vi "Joystick and Camera SHIH V5- external Connection.vi"(0 "Motion in":refnum<class "Motion.lvclass">, 1 "XYZTheta":dbl[](array[numeric])=[584.964, 676.042, 69.3079, 0.000384], 2 "Measurement Point":string, 3 "Inital GO":bool=TRUE) -> (5 "final out":dbl[](array[numeric]), 7 "Motion out":refnum<class "Motion.lvclass">, 10 "error out":errorcluster)   [LabVIEW 2016]
uses:
  Classes/Controllers/Motion/Copy of Motion Folder/Motion.lvclass
panel:
  in  "how many times per measurement":dbl=50.0
  out "Gantry position":dbl[](array[numeric])
  in  "start measurement":bool
  in  "Joystick":bool
  in  "Stop":bool
  # "new world"
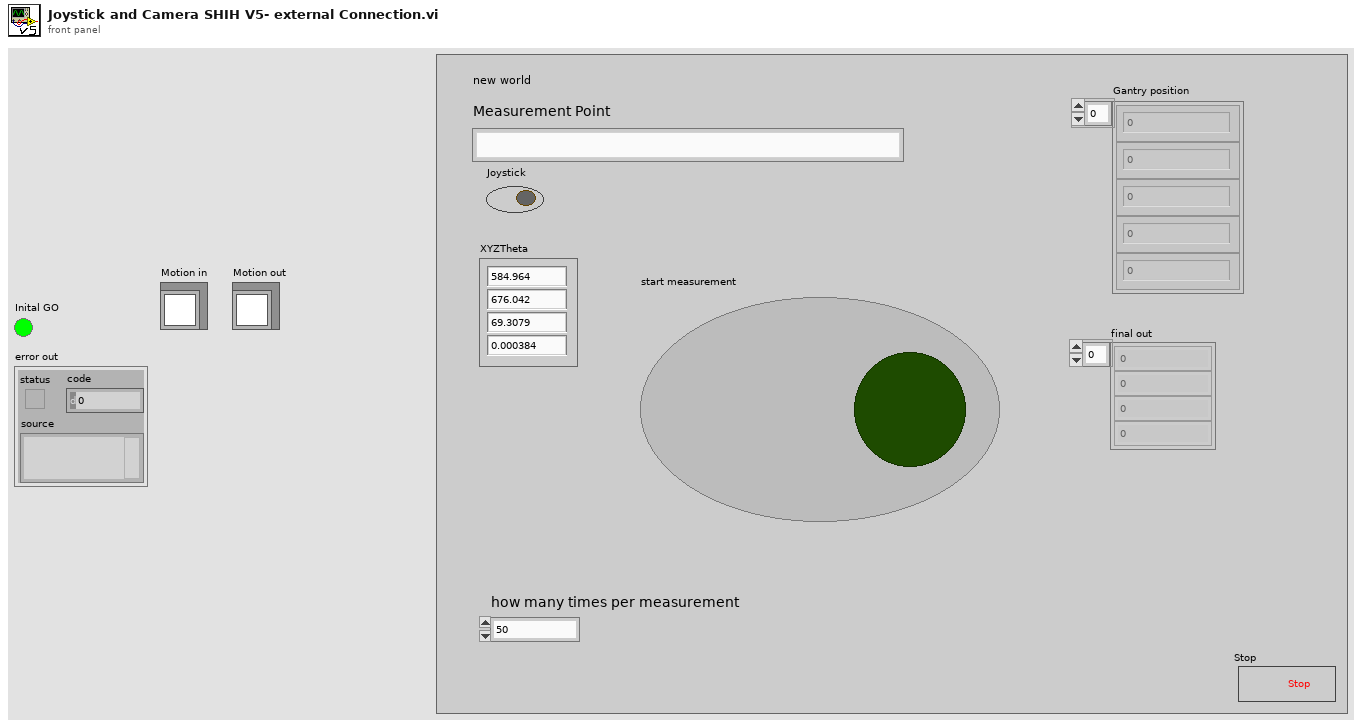
[diagram p1: front panel]
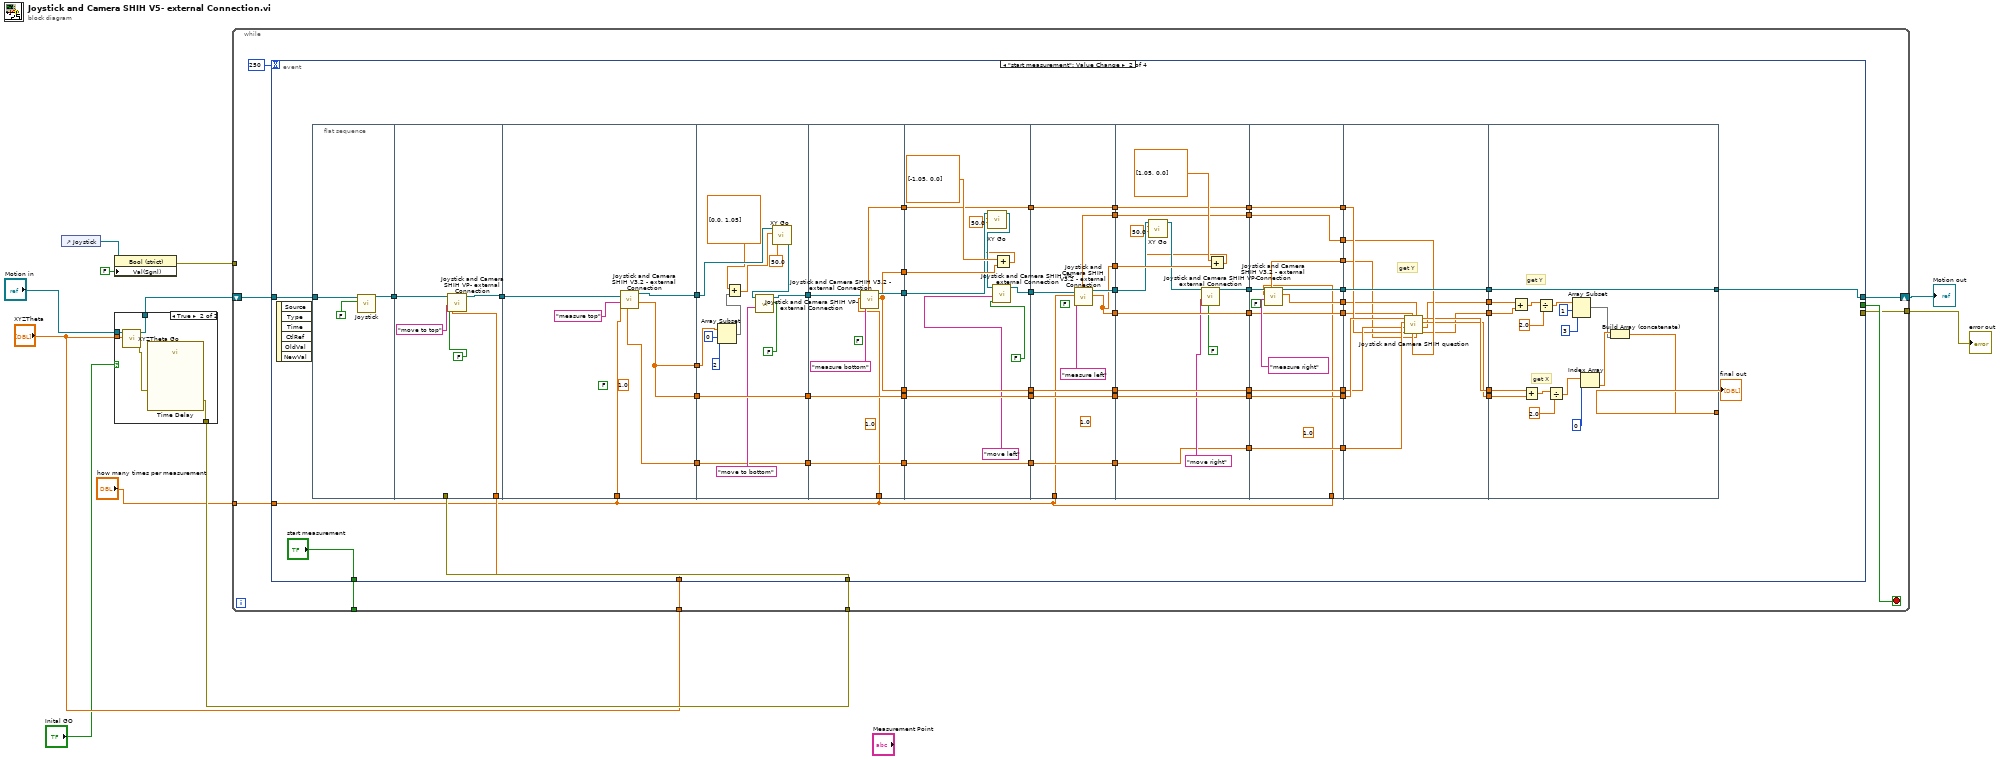
[diagram p0: block diagram]
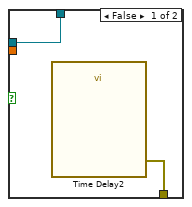
[diagram p2: hidden frame]
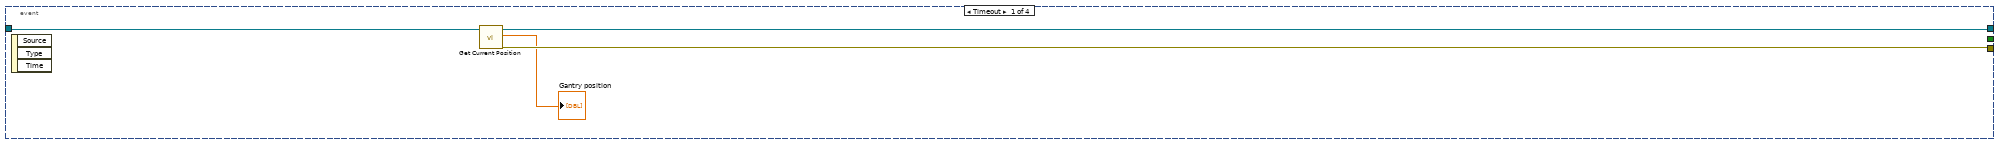
[diagram p3: hidden frame]
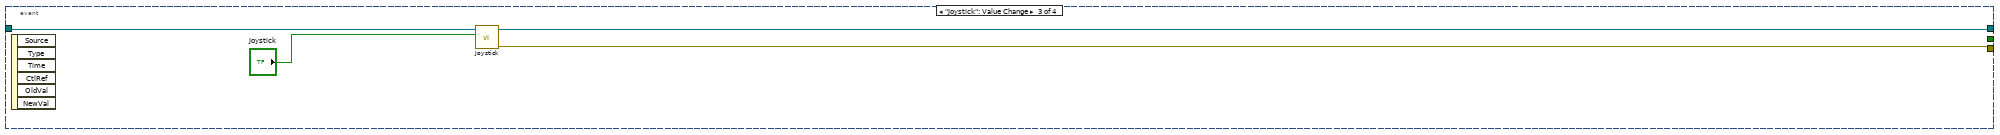
[diagram p4: hidden frame]
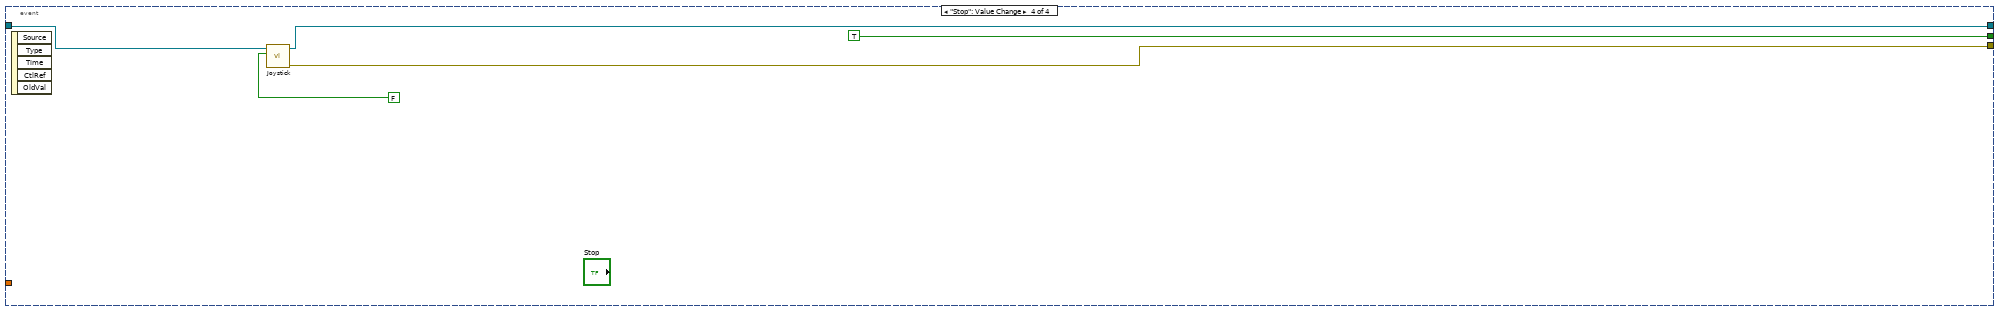
[diagram p5: hidden frame]
diagram:
  n1 = control-ref of="Joystick"() -> (w10:refnum<vi>)
  n2 = case shown="True" "Inital GO" {
    tunnel: "Motion in" -> [w13 w18]
    tunnel: [w13 w17] -> w5
    tunnel: [w12 w15] -> w4
    tunnel: "XYZTheta" -> [_ w14]
    frame False {
      n3 = call "Time Delay2"() -> ("error out"=w12:errorcluster)  [unwired: 11 in]
    }
    frame True {
      n4 = call "XYZTheta Go.vi"("XYZTheta In"=w14, "Motion in"=w18) -> ("error out"=w16:errorcluster, "Motion out"=w17:refnum<class "Motion.lvclass">)  [unwired: 7 in, 1 out]
      n5 = call "Time Delay"("error in (no error)"=w16) -> ("error out"=w15:errorcluster)  [unwired: 10 in]
    }
  }
  n6 = property class="Bool (strict)"(reference=w10, "Val(Sgnl)"=FALSE ("Value (Signaling)")) -> (error out=w9:errorcluster)  [unwired: 1 in, 1 out]
  n7 = while {
    shift-right: [w24] -> w8
    shift-left: w5 -> [w25]
    tunnel: w9 -> [_]
    tunnel: [w23] -> w7
    tunnel: w4 -> [w22]
    tunnel: "XYZTheta" -> [w21]
    tunnel: [w20] -> _
    tunnel: "how many times per measurement" -> [w19]
    stop <- w26 stop-if-true
    n8 = event shown="[1] \"start measurement\": Value Change" {
      selector: _ -> [_ _ _ _]
      dyn-events: _ -> [_ _ _ _]
      timeout: 250 -> [_ _ _ _]
      tunnel: [_ _ _ TRUE] -> w26
      tunnel: w25 -> [w31 w87 w207 w211]
      tunnel: [w30 w62 w205 w210] -> w24
      tunnel: [w29 _ w204 w208] -> w23
      tunnel: w22 -> [_ w86 _ _]
      tunnel: w21 -> [_ w64 _ _]
      tunnel: [_ "start measurement" _ _] -> w20
      tunnel: w19 -> [_ w32 _ _]
      event Timeout {
        n9 = event-data() -> ()  [unwired: 1 in, 3 out]
        n10 = call-dynamic "Get Current Position.vi"("Motion in"=w31) -> ("error out"=w29:errorcluster, "XYZTheta Out"=→"Gantry position":dbl[], "Motion out"=w30:refnum<class "Motion.lvclass">)  [unwired: 8 in]
      }
      event "start measurement": Value Change {
        n11 = event-data() -> ()  [unwired: 1 in, 6 out]
        n12 = flat-sequence {
          tunnel: w87 -> [w89]
          tunnel: [w88] -> w84
          tunnel: w86 -> [_]
          tunnel: [w91] -> w85
          tunnel: w84 -> [w95]
          tunnel: w64 -> [w92]
          tunnel: w85 -> [w101]
          tunnel: [w100] -> w83
          tunnel: [w98] -> w72
          tunnel: [w98] -> w61
          tunnel: [w97] -> w48
          tunnel: w32 -> [w96]
          tunnel: w83 -> [w111]
          tunnel: [w114] -> w82
          tunnel: [w115] -> w73
          tunnel: w72 -> [w115]
          tunnel: w61 -> [w106]
          tunnel: w48 -> [w102]
          tunnel: [w102] -> w47
          tunnel: w82 -> [w123]
          tunnel: [w121] -> w81
          tunnel: [w120] -> w74
          tunnel: w73 -> [w120]
          tunnel: [w119] -> w68
          tunnel: [w119] -> w60
          tunnel: w47 -> [w118]
          tunnel: [w118] -> w46
          tunnel: [w117] -> w41
          tunnel: w32 -> [w116]
          tunnel: w81 -> [w129]
          tunnel: [w134] -> w80
          tunnel: [w136] -> w75
          tunnel: w74 -> [w136]
          tunnel: [w135] -> w69
          tunnel: w68 -> [w135]
          tunnel: w60 -> [w130]
          tunnel: w46 -> [w125]
          tunnel: [w125] -> w45
          tunnel: w41 -> [w124]
          tunnel: [w124] -> w40
          tunnel: w80 -> [w146]
          tunnel: [w145] -> w79
          tunnel: [w143] -> w76
          tunnel: w75 -> [w143]
          tunnel: [w142] -> w70
          tunnel: w69 -> [w142]
          tunnel: [w141] -> w66
          tunnel: [w141] -> w59
          tunnel: w45 -> [w140]
          tunnel: [w140] -> w44
          tunnel: w40 -> [w139]
          tunnel: [w139] -> w39
          tunnel: [w138] -> w36
          tunnel: w32 -> [w137]
          tunnel: w79 -> [w153]
          tunnel: [w158] -> w78
          tunnel: [w161] -> w77
          tunnel: w76 -> [w161]
          tunnel: [w160] -> w71
          tunnel: w70 -> [w160]
          tunnel: [w159] -> w67
          tunnel: w66 -> [w159]
          tunnel: w59 -> [w154]
          tunnel: w44 -> [w149]
          tunnel: [w149] -> w43
          tunnel: w39 -> [w148]
          tunnel: [w148] -> w38
          tunnel: w36 -> [w147]
          tunnel: [w147] -> w35
          tunnel: w78 -> [w173]
          tunnel: [w171] -> w58
          tunnel: w77 -> [w171]
          tunnel: [w170] -> w56
          tunnel: w71 -> [w170]
          tunnel: [w169] -> w54
          tunnel: [w168] -> w52
          tunnel: w67 -> [w168]
          tunnel: [w167] -> w50
          tunnel: w43 -> [w166]
          tunnel: [w166] -> w42
          tunnel: w38 -> [w165]
          tunnel: [w165] -> w37
          tunnel: w35 -> [w164]
          tunnel: [w164] -> w34
          tunnel: [w163] -> w33
          tunnel: w32 -> [w162]
          tunnel: w58 -> [w185]
          tunnel: [w176] -> w57
          tunnel: w56 -> [w183]
          tunnel: [w177] -> w55
          tunnel: w54 -> [w179]
          tunnel: [w175] -> w53
          tunnel: w52 -> [w181]
          tunnel: [w174] -> w51
          tunnel: w50 -> [w186]
          tunnel: [w186] -> w49
          tunnel: w42 -> [w184]
          tunnel: w37 -> [w182]
          tunnel: w34 -> [w180]
          tunnel: w33 -> [w178]
          tunnel: w57 -> [w203]
          tunnel: w55 -> [w202]
          tunnel: w53 -> [w197]
          tunnel: w51 -> [w196]
          tunnel: [w188] -> w63
          tunnel: w49 -> [w187]
          tunnel: [w187] -> w62
          frame #0 {
            n13 = call-dynamic "Joystick.vi"("Joystick"=FALSE, "Motion in"=w89) -> ("Motion out"=w88:refnum<class "Motion.lvclass">)  [unwired: 8 in, 1 out]
          }
          frame #1 {
            n14 = call "Joystick and Camera SHIH VP- external Connection.vi"("Motion in"=w95, "XYZTheta"=w92, "Measurement Point"="move to top", "Inital GO"=FALSE) -> ("Motion out"=w91:refnum<class "Motion.lvclass">)  [unwired: 3 in, 3 out]
          }
          frame #2 {
            (unwired) 1.0 ("reset the counting")
            (unwired) FALSE ("Inital GO")
            n15 = call "Joystick and Camera SHIH V3.2 - external Connection.vi"("Measurement Point"="measure top", "times per measurement"=w96, "Motion in"=w101) -> ("final out"=w98:dbl[], "Motion out 2"=w100:refnum<class "Motion.lvclass">, "radius/stddev"=w97:dbl[])  [unwired: 2 in, 2 out]
          }
          frame #3 {
            n16 = Array Subset(array=w106, index=0, length=2) -> (w104:dbl[])
            n17 = Add(x=dbl[] [0.0, 1.05], y=w104) -> (x+y=w103:dbl[])
            n18 = call-dynamic "XY Go.vi"("Speed"=50.0, "XY"=w103, "Motion in"=w111) -> ("Motion out"=w110:refnum<class "Motion.lvclass">)  [unwired: 7 in, 1 out]
            n19 = call "Joystick and Camera SHIH VP- external Connection.vi"("Motion in"=w110, "Measurement Point"="move to bottom", "Inital GO"=FALSE) -> ("Motion out"=w114:refnum<class "Motion.lvclass">)  [unwired: 4 in, 3 out]
          }
          frame #4 {
            (unwired) 1.0 ("reset the counting")
            (unwired) FALSE ("Inital GO")
            n20 = call "Joystick and Camera SHIH V3.2 - external Connection.vi"("Measurement Point"="measure bottom", "times per measurement"=w116, "Motion in"=w123) -> ("final out"=w119:dbl[], "Motion out 2"=w121:refnum<class "Motion.lvclass">, "radius/stddev"=w117:dbl[])  [unwired: 2 in, 2 out]
          }
          frame #5 {
            n21 = Add(x=dbl[] [-1.05, 0.0], y=w130) -> (x+y=w127:dbl[])
            n22 = call-dynamic "XY Go.vi"("Speed"=50.0, "XY"=w127, "Motion in"=w129) -> ("Motion out"=w128:refnum<class "Motion.lvclass">)  [unwired: 7 in, 1 out]
            n23 = call "Joystick and Camera SHIH VP- external Connection.vi"("Motion in"=w128, "Measurement Point"="move left", "Inital GO"=FALSE) -> ("Motion out"=w134:refnum<class "Motion.lvclass">)  [unwired: 4 in, 3 out]
          }
          frame #6 {
            (unwired) 1.0 ("reset the counting")
            (unwired) FALSE ("Inital GO")
            n24 = call "Joystick and Camera SHIH V3.2 - external Connection.vi"("Measurement Point"="measure left", "times per measurement"=w137, "Motion in"=w146) -> ("final out"=w141:dbl[], "Motion out 2"=w145:refnum<class "Motion.lvclass">, "radius/stddev"=w138:dbl[])  [unwired: 2 in, 2 out]
          }
          frame #7 {
            n25 = Add(x=dbl[] [1.05, 0.0], y=w154) -> (x+y=w151:dbl[])
            n26 = call-dynamic "XY Go.vi"("Speed"=50.0, "XY"=w151, "Motion in"=w153) -> ("Motion out"=w152:refnum<class "Motion.lvclass">)  [unwired: 7 in, 1 out]
            n27 = call "Joystick and Camera SHIH VP- external Connection.vi"("Motion in"=w152, "Measurement Point"="move right", "Inital GO"=FALSE) -> ("Motion out"=w158:refnum<class "Motion.lvclass">)  [unwired: 4 in, 3 out]
          }
          frame #8 {
            (unwired) 1.0 ("reset the counting")
            (unwired) FALSE ("Inital GO")
            n28 = call "Joystick and Camera SHIH V3.2 - external Connection.vi"("Measurement Point"="measure right", "times per measurement"=w162, "Motion in"=w173) -> ("final out"=w169:dbl[], "Motion out 2"=w167:refnum<class "Motion.lvclass">, "radius/stddev"=w163:dbl[])  [unwired: 2 in, 2 out]
          }
          frame #9 {
            # "get Y"
            n29 = call "Joystick and Camera SHIH question.vi"("right Std dev"=w178, "right final out"=w179, "left Std dev"=w180, "left final out"=w181, "down Std dev"=w182, "down final out"=w183, "up Std dev"=w184, "up final out"=w185) -> ("Y 1"=w174:dbl[], "Y 2"=w175:dbl[], "X 2"=w176:dbl[], "X 1"=w177:dbl[])
          }
          frame #10 {
            # "get X"
            # "get Y"
            n30 = Add(x=w197, y=w196) -> (x+y=w198:dbl[])
            n31 = Add(x=w202, y=w203) -> (x+y=w200:dbl[])
            n32 = Divide(x=w198, y=2.0) -> (x/y=w193:dbl[])
            n33 = Divide(x=w200, y=2.0) -> (x/y=w195:dbl[])
            n34 = Array Subset(array=w193, index=1, length=3) -> (w189:dbl[])
            n35 = Index Array(array=w195, index=0) -> (element=w190:dbl)
            n36 = Build Array (concatenate)(w190, w189) -> (w188:dbl[])
          }
        }
        "final out" <- w63
      }
      event "Joystick": Value Change {
        n37 = event-data() -> ()  [unwired: 1 in, 6 out]
        n38 = call-dynamic "Joystick.vi"("Joystick"="Joystick", "Motion in"=w207) -> ("error out"=w204:errorcluster, "Motion out"=w205:refnum<class "Motion.lvclass">)  [unwired: 8 in]
      }
      event "Stop": Value Change {
        n39 = event-data() -> ()  [unwired: 1 in, 5 out]
        n40 = call-dynamic "Joystick.vi"("Joystick"=FALSE, "Motion in"=w211) -> ("error out"=w208:errorcluster, "Motion out"=w210:refnum<class "Motion.lvclass">)  [unwired: 8 in]
      }
    }
  }
  "error out" <- w7
  "Motion out" <- w8
